vi "New.vi"(4 "Unescaped":bool, 6 "Delimiters":cluster{"Close":string, "Open":string}={"Close"="}}", "Open"="{{"}, 8 "Error In":errorcluster, 11 "Key":string) -> (0 "Error Out":errorcluster, 3 "Tag":refnum<class "Tag.lvclass">)   [LabVIEW 2018, in "Toolkit.lvlib" / "Nodes.lvlib" / "Tag.lvclass"]
uses:
  Tag.lvclass
  Tag.lvclass/Tag.ctl
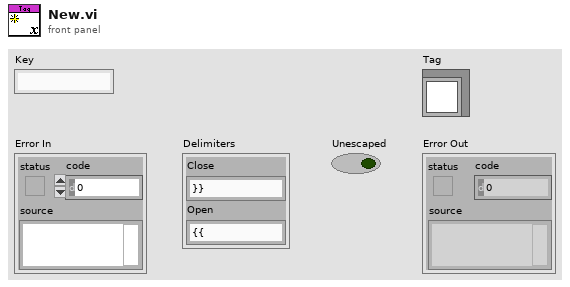
[diagram p1: front panel]
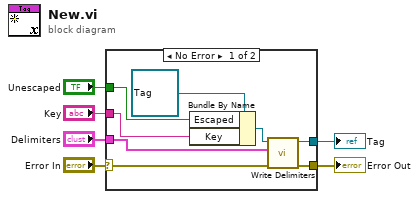
[diagram p0: block diagram]
diagram:
  n1 = case shown="No Error" "Error In" {
    selector: "Error In" -> [w7 w15]
    tunnel: "Key" -> [w14 _]
    tunnel: "Unescaped" -> [w13 _]
    tunnel: [w10 _] -> w4
    tunnel: [w9 w15] -> w3
    tunnel: "Delimiters" -> [w8 _]
    frame No Error {
      n2 = Bundle By Name(cluster=refnum<class "Tag.lvclass"> refnum ("Toolkit.lvlib:Nodes.lvlib:EscapedTag.lvclass"), "Escaped"=w13, "Key"=w14) -> (w12:refnum<class "Tag.lvclass">)
      n3 = call-dynamic "Write Delimiters.vi"("Error In"=w7, "Delimiters"=w8, "Node In"=w12) -> ("Error Out"=w9:errorcluster, "Node Out"=w10:refnum<class "Tag.lvclass">)  [unwired: 7 in]
    }
    frame Error {
    }
  }
  "Tag" <- w4
  "Error Out" <- w3
